vi "Destriy Events.vi"(8 "error in (no error)":errorcluster, 11 "Task Viewer in":refnum<class "Task Viewer.lvclass">) -> (0 "error out":errorcluster, 3 "Task Viewer out":refnum<class "Task Viewer.lvclass">)   [LabVIEW 2020, in "Task Viewer.lvlib" / "Task Viewer.lvclass"]
uses:
  Task Viewer.lvclass
  Task Viewer.lvclass/Task Viewer.ctl
panel:
  out "error out 2":errorcluster
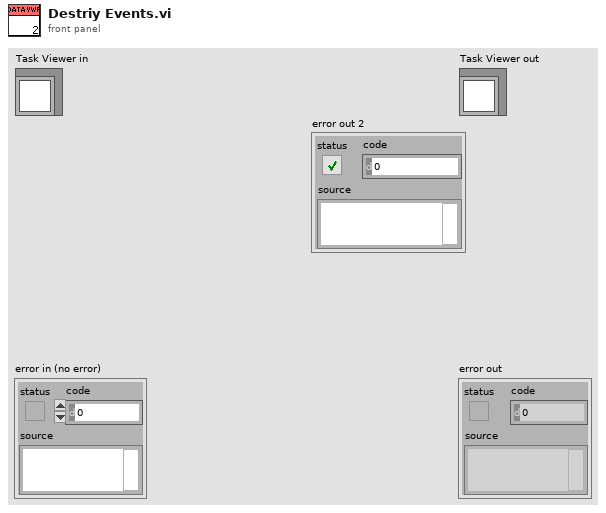
[diagram p1: front panel]
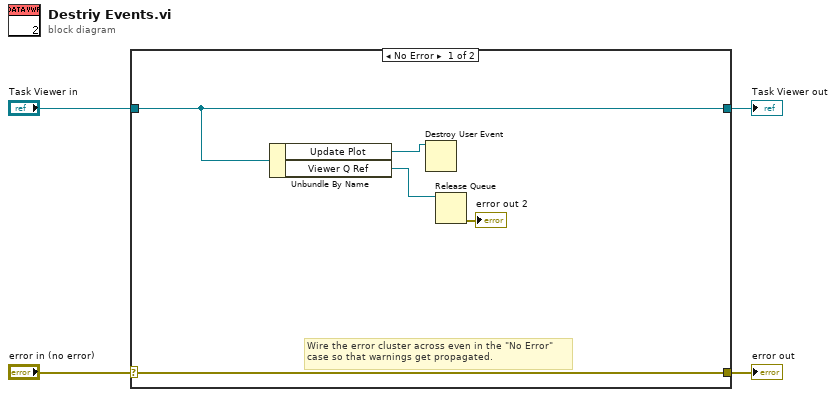
[diagram p0: block diagram]
diagram:
  n1 = case shown="No Error" "error in (no error)" {
    selector: "error in (no error)" -> [w9 w11]
    tunnel: [w9 w11] -> w3
    tunnel: [w8 w10] -> w1
    tunnel: "Task Viewer in" -> [w8 w10]
    frame No Error {
      # "Wire the error cluster across even in the \"No Error\"\ncase so that warnings get propagated."
      n2 = Unbundle By Name(w8) -> ("Update Plot"=w7:refnum<user-event>, "Viewer Q Ref"=w6:refnum<queue>)
      n3 = Destroy User Event(user event=w7) -> ()  [unwired: 1 in, 1 out]
      n4 = Release Queue(queue=w6) -> (error out=→"error out 2":errorcluster)  [unwired: 2 in, 2 out]
    }
    frame Error {
    }
  }
  "error out" <- w3
  "Task Viewer out" <- w1
